vi "get Texture.vi"(11 "Texture Name":string) -> (3 "Texture":refnum<class "Texture.lvclass">)   [LabVIEW 2021, in "Resource Manager.lvclass"]
uses:
  Resource Manager.lvclass
  Texture/Texture.lvclass
  Resource Manager.lvclass/Resource Manager.ctl
  Globals.vi
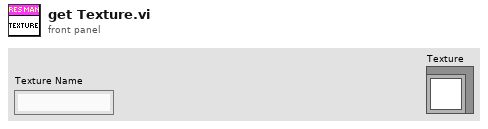
[diagram p1: front panel]
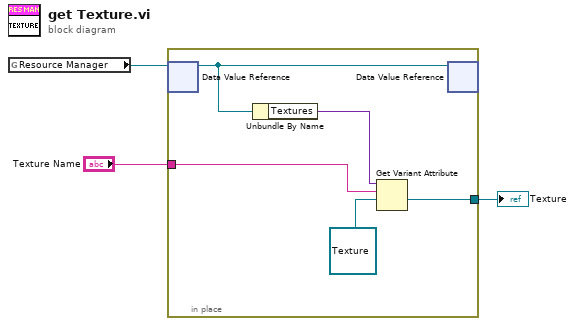
[diagram p0: block diagram]
diagram:
  n1 = global read "Globals.vi" "Resource Manager"() -> (w1:refnum<data-value>)
  n2 = in-place {
    in-place-border: "Texture Name" -> [w8]
    in-place-border: [w6] -> w2
    n3 = in-place-dvr #1(w1) -> (w4:refnum<class "Resource Manager.lvclass">)  [unwired: 1 out]
    n4 = Unbundle By Name(w4) -> ("Textures"=w5:variant)
    n5 = Get Variant Attribute(Variant=w5, name=w8, default value (empty Variant)=refnum<class "Texture.lvclass"> refnum ("Texture in")) -> (value=w6:refnum<class "Texture.lvclass">)  [unwired: 1 in, 3 out]
    n6 = in-place-dvr #1(w4) -> ()  [unwired: 2 out]
  }
  "Texture" <- w2
